vi "runSettingsBackEnd.vi"(8 "error in (no error)":errorcluster, 11 "CameraManager in":refnum<class "CameraManager.lvclass">) -> (0 "error out":errorcluster)   [LabVIEW 2011, in "iManagement.lvlib" / "CameraManager.lvclass"]
uses:
  CameraManager.lvclass
  CameraManager.lvclass/CameraManager.ctl
  Hal/Channels/Camera/CameraController.lvclass
  Tools/SettingsManager/SettingsManager.lvclass
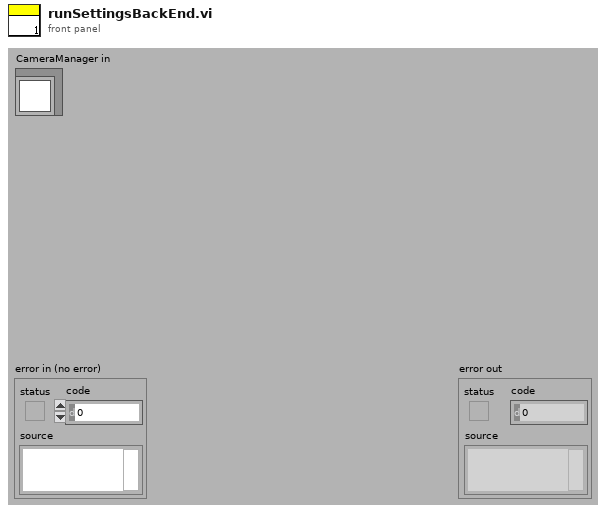
[diagram p1: front panel]
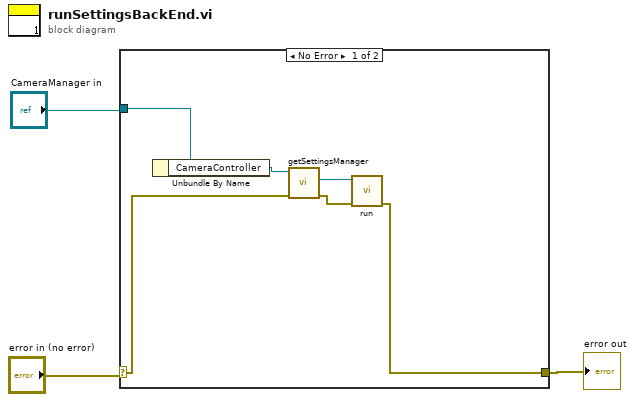
[diagram p0: block diagram]
diagram:
  n1 = case shown="No Error" "error in (no error)" {
    selector: "error in (no error)" -> [w7 w10]
    tunnel: [w4 w10] -> w3
    tunnel: "CameraManager in" -> [w9 _]
    frame No Error {
      n2 = Unbundle By Name(w9) -> ("CameraController"=w8:refnum<class "CameraController.lvclass">)
      n3 = call-dynamic "getSettingsManager.vi"("error in (no error)"=w7, "CameraController.lvclass in"=w8) -> ("error out"=w5:errorcluster, "Tools.lvlib:Settings.lvlib:SettingsManager.lvclass"=w6:refnum<class "SettingsManager.lvclass">)  [unwired: 7 in, 1 out]
      n4 = call-dynamic "run.vi"("error in (no error)"=w5, "SettingsManager in"=w6) -> ("error out"=w4:errorcluster)  [unwired: 8 in, 1 out]
    }
    frame Error {
    }
  }
  "error out" <- w3
